vi "Modbus Write U16.vi"(7 "Slave Address":u8, 8 "error in (no error)":errorcluster, 9 "Input data U16":u16, 10 "Register Start Address":u16 format="%x", 11 "VISA resource in":refnum<visa-resource-name>) -> (0 "error out":errorcluster, 3 "VISA resource out":refnum<visa-resource-name>)   [LabVIEW 2024, in "Voegtlin_NI_SMART_Modbus_Drivers.lvlib"]
doc: "Schreibe einen U16-Wert an die angegebene des selektierten Geraetes.\nDer COM-Port muss dazu initialisiert sein (benutze\" Modbus Init.vi\")."
uses:
  Voegtlin_NI_SMART_Modbus_Drivers.lvlib
  Enums/Modbus Comm.ctl
panel:
  out "U16 input data to write\n(array)":u16[](array[numeric])
  # "Input Data"
  # "Internal Data"
  # "Output Data"
  # "(Inputmaske in HEX)"
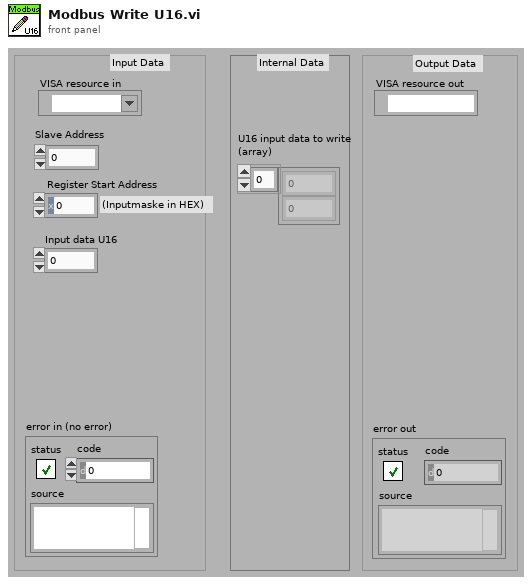
[diagram p1: front panel]
types:
  T1 = typedef "Voegtlin_NI_SMART_Modbus_Drivers.lvlib/Modbus Comm.ctl" = enum16{"Init", "Read", "Write", "Exit"}
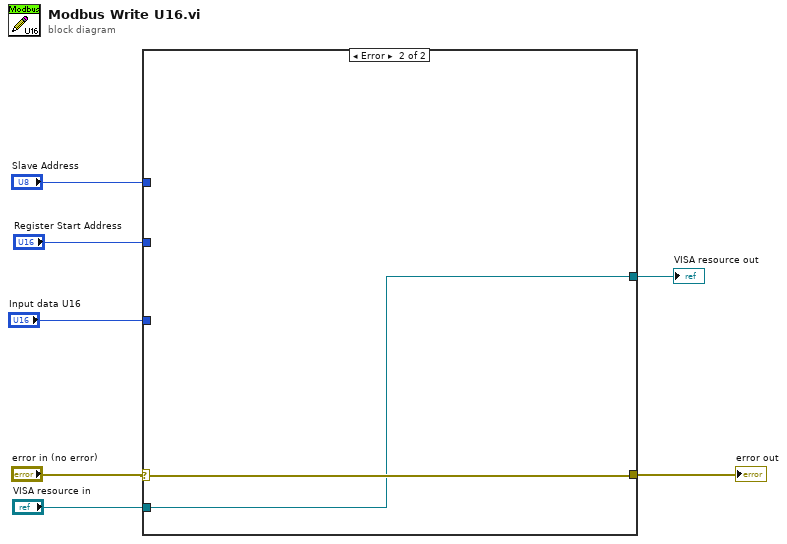
[diagram p0: block diagram]
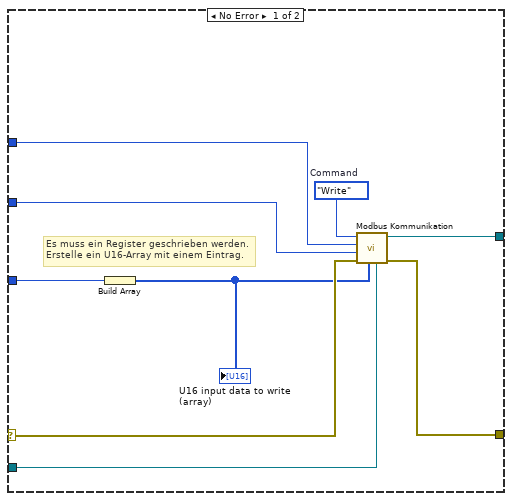
[diagram p2: hidden frame]
diagram:
  n1 = case shown="Error" "error in (no error)" {
    selector: "error in (no error)" -> [w13 w18]
    tunnel: "Register Start Address" -> [w11 _]
    tunnel: [w16 w18] -> w6
    tunnel: "Input data U16" -> [w14 _]
    tunnel: "Slave Address" -> [w10 _]
    tunnel: "VISA resource in" -> [w9 w17]
    tunnel: [w8 w17] -> w1
    frame No Error {
      w15 = Modbus_Comm."Write"  # Command
      # "Es muss ein Register geschrieben werden. Erstelle ein U16-Array mit einem Eintrag."
      n2 = Build Array(w14) -> (w12:u16[])
      "U16 input data to write\n(array)" <- w12
      n3 = call "Modbus Kommunikation.vi"("VISA resource in"=w9, "Data In / #Reads [U16]"=w12, "error in (no error)"=w13, "Register Start Address"=w11, "Slave Address"=w10, "Command"=w15) -> ("error out"=w16:errorcluster, "VISA resource out"=w8:refnum<visa-resource-name>)  [unwired: 3 in, 1 out]
    }
    frame Error {
    }
  }
  "error out" <- w6
  "VISA resource out" <- w1
